vi "读取AVI文件V1（简化版）.vi"() -> ()   [LabVIEW 2013]
panel:
  out "x-y":u32
  in  "value":bool
  in  "milliseconds to wait":u32=100
  in  "AVI File Path":path
  out "Image":T1(plugin-control)
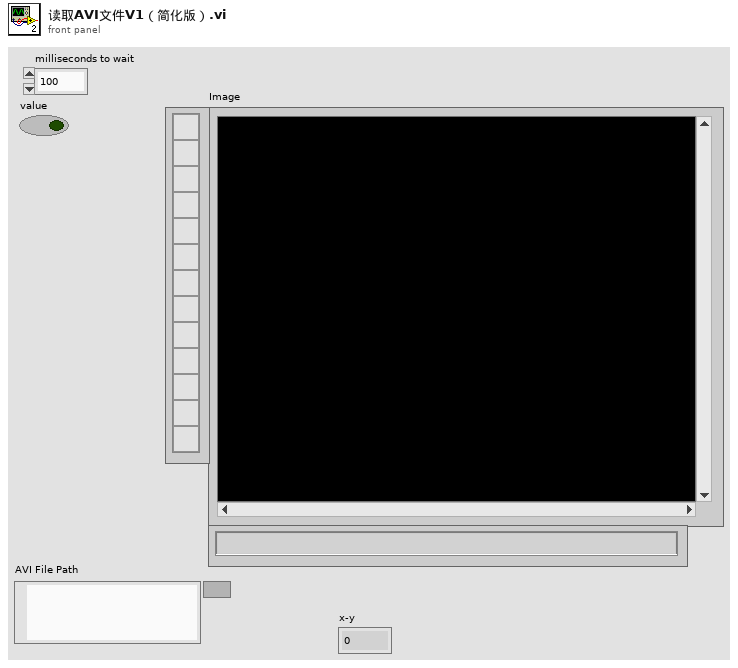
[diagram p1: front panel]
types:
  T1 = typedef "IMAQ Image.ctl" = refnum<image>
  T2 = typedef "AviRefnum.ctl" = refnum<k1>
  T3 = typedef "Image Type" = u32
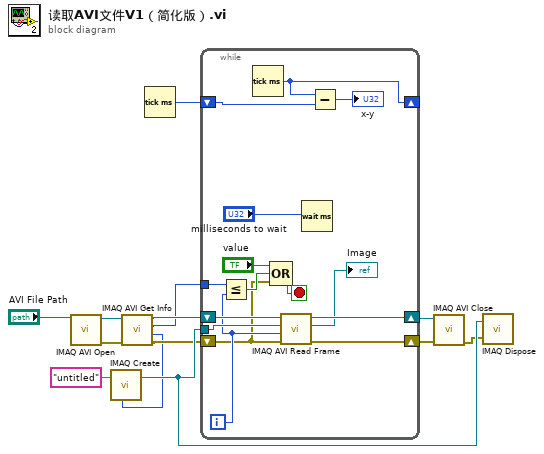
[diagram p0: block diagram]
diagram:
  n1 = call "IMAQ AVI Open"("AVI Path"="AVI File Path") -> ("error out"=w9:errorcluster, "Avi Refnum"=w10:T2)  [unwired: 1 in, 8 out]
  n2 = call "IMAQ AVI Get Info"("error in (no error)"=w9, "Avi Refnum"=w10) -> ("error out"=w7:errorcluster, "Image Type"=w1:T3, "Number of Frames"=w6:u32, "Avi Refnum (duplicate)"=w8:T2)  [unwired: 6 out]
  n3 = call "IMAQ Create"("Image Name"="untitled", "Image Type"=w1) -> ("New Image"=w13:T1)  [unwired: 3 in, 1 out]
  n4 = Tick Count (ms)() -> (millisecond timer value=w2:u32)
  n5 = while {
    tunnel: w6 -> [w28]
    tunnel: w13 -> [w25]
    shift-right: [w22] -> w4
    shift-left: w8 -> [w26]
    shift-right: [w23] -> w5
    shift-left: w7 -> [w18]
    shift-right: [w15] -> _
    shift-left: w2 -> [w16]
    i -> [w24]
    stop <- w19 stop-if-true
    n6 = Less Or Equal?(x=w28, y=w24) -> (x <= y?=w20:bool)
    n7 = Tick Count (ms)() -> (millisecond timer value=w15:u32)
    n8 = Compound Arithmetic op=OR("value", w20, w18) -> (w19:bool)
    n9 = call "IMAQ AVI Read Frame"("error in (no error)"=w18, "Frame Number"=w24, "Image"=w25, "Avi Refnum"=w26) -> ("error out"=w23:errorcluster, "Image Out"=→"Image":T1, "Avi Refnum (duplicate)"=w22:T2)  [unwired: 1 in, 4 out]
    n10 = Wait (ms)(milliseconds to wait="milliseconds to wait") -> ()  [unwired: 1 out]
    n11 = Subtract(x=w15, y=w16) -> (x-y=→"x-y":u32)
  }
  n12 = call "IMAQ AVI Close"("error in (no error)"=w5, "Avi Refnum"=w4) -> ("error out"=w3:errorcluster)  [unwired: 9 out]
  n13 = call "IMAQ Dispose"("Image"=w13, "error in (no error)"=w3) -> ()  [unwired: 4 in, 1 out]
